vi "Get VI Description.vi"() -> ()   [LabVIEW 2012, in "Application.lvlib"]
uses:
  Application.lvlib
panel:
  out "错误输出":errorcluster
  in  "错误输入（无错误）":errorcluster
  out "VI Description":string
  in  "VI Path":path
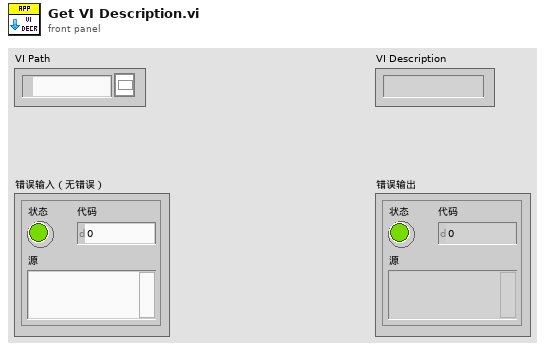
[diagram p1: front panel]
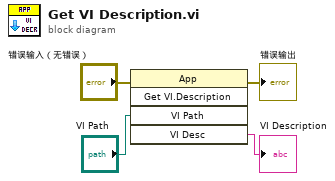
[diagram p0: block diagram]
diagram:
  n1 = invoke class="App" method="Get VI.Description"(error in="错误输入（无错误）", "VI Path"="VI Path") -> (error out=→"错误输出":errorcluster, "VI Desc"=→"VI Description":string)  [unwired: 3 in, 3 out]
